vi "ConfigureRobot.vi"(8 "Pigeon Talon":T1, 9 "Pigeon":T6 {"Type" items=["CAN"=352321536, "TalonSRX"=33554432]}, 10 "Right Side":T1, 11 "Left Side":T1) -> (1 "Pigeon":T6 {"Type" items=["CAN"=352321536, "TalonSRX"=33554432]}, 2 "Right Side":T1, 3 "Left Side":T1)   [LabVIEW 2017]
uses:
  <vilib>/Rock Robotics/WPI/ThirdParty/Phoenix-LabVIEW/Pigeon IMU/CTRE_PigeonIMU_DeviceRef.ctl
  <vilib>/Rock Robotics/WPI/ThirdParty/Phoenix-LabVIEW/Pigeon IMU/CTRE_PigeonIMU_ConnectionType.ctl
  <vilib>/Rock Robotics/WPI/MotorControl/WPI_MotorControlDeviceRef.ctl
  <vilib>/Rock Robotics/WPI/MotorControl/WPI_MotorControlType.ctl
  <vilib>/Rock Robotics/SystemInterfaces/DIO/FPGA_DIOPWMChannel.ctl
  <vilib>/Rock Robotics/WPI/PWM/WPI_PWMDeadband.ctl
  <vilib>/Rock Robotics/SystemInterfaces/DIO/FPGA_DIOChannel.ctl
  <vilib>/Rock Robotics/WPI/ThirdParty/Phoenix-LabVIEW/Motor Controller/Controls/CTRE_Phoenix_MotorControl_FeedbackDevice.ctl
  <vilib>/Rock Robotics/WPI/ThirdParty/Phoenix-LabVIEW/Motor Controller/Controls/CTRE_Phoenix_MotorControl_RemoteSourceType.ctl
  <vilib>/Rock Robotics/WPI/ThirdParty/Phoenix-LabVIEW/Motor Controller/Controls/CTRE_Phoenix_MotorControl_SensorTermFeedbackDevice_Enhanced.ctl
  <vilib>/Rock Robotics/WPI/ThirdParty/Phoenix-LabVIEW/Motor Controller/Controls/CTRE_Phoenix_MotorControl_StatusFrameEnhanced.ctl
  <vilib>/Rock Robotics/WPI/ThirdParty/Phoenix-LabVIEW/Motor Controller/Controls/CTRE_Phoenix_MotorControl_NeutralMode.ctl
  <vilib>/Rock Robotics/WPI/ThirdParty/Phoenix-LabVIEW/Motor Controller/Controls/CTRE_Phoenix_MotorControl_ControlMode.ctl
  Constants.vi
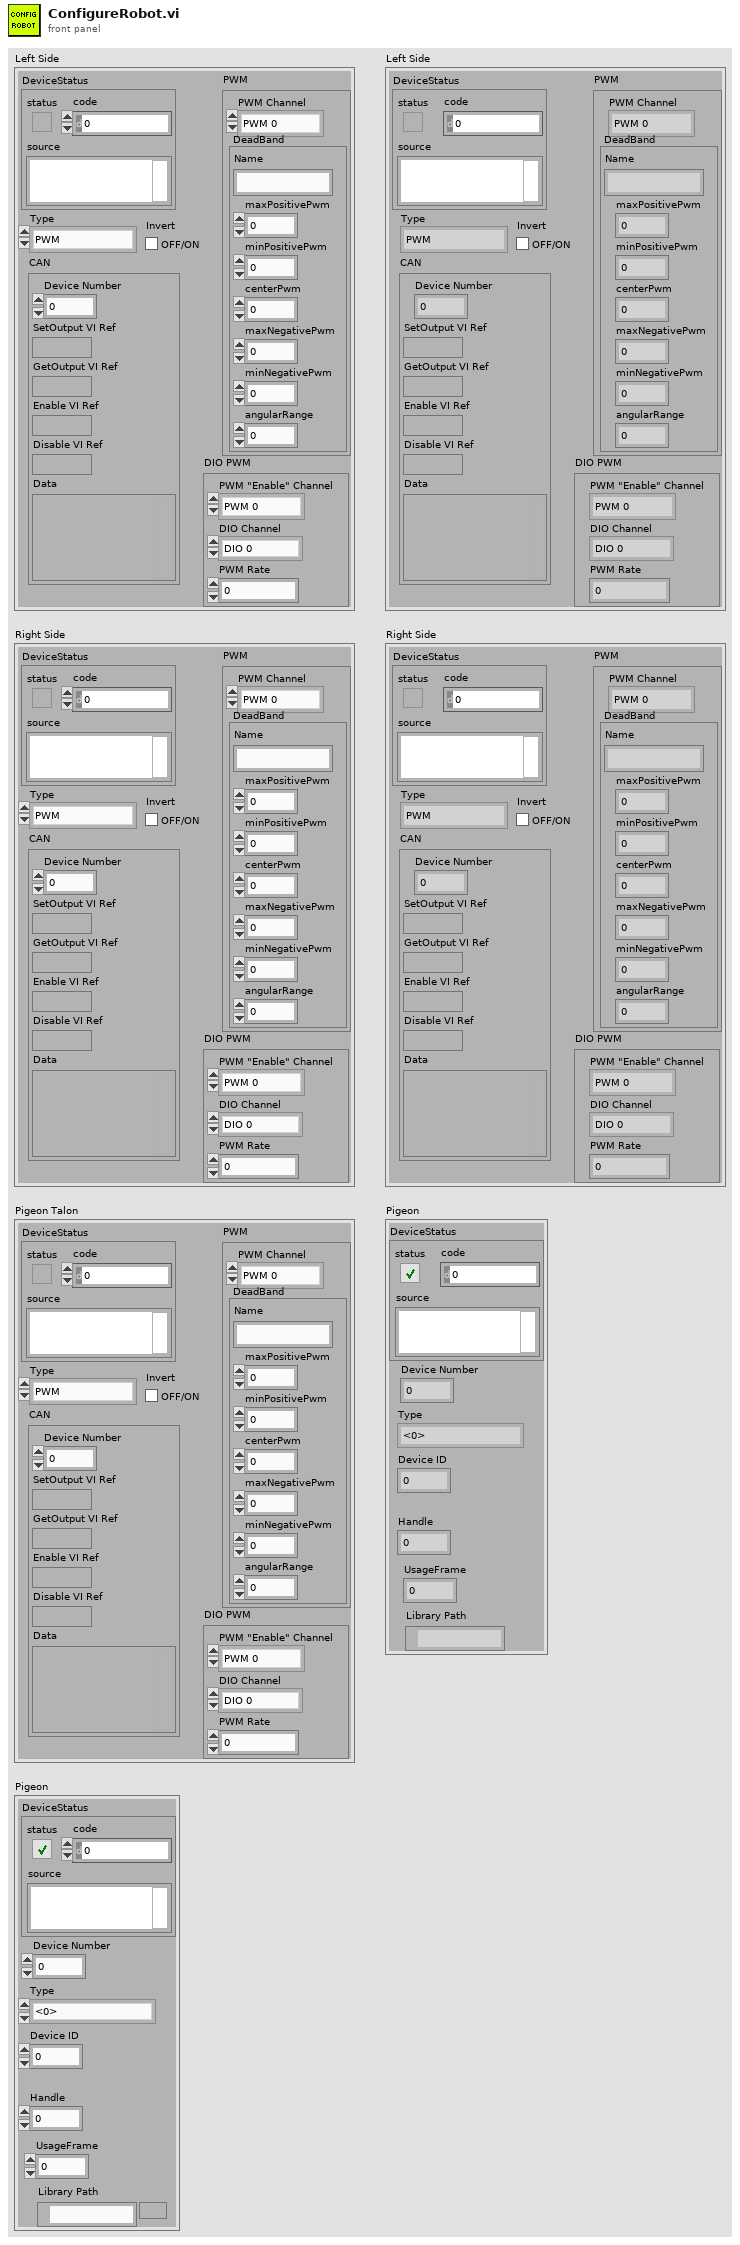
[diagram p1: front panel]
types:
  T1 = typedef "WPI_MotorControlDeviceRef.ctl" = cluster{"DeviceStatus":errorcluster, "Type":T2, "PWM":cluster{"PWM Channel":T3, "DeadBand":T4}, "CAN":cluster{"Device Number":u8, "SetOutput VI Ref":variant, "GetOutput VI Ref":variant, "Enable VI Ref":variant, "Disable VI Ref":variant, "Data":variant}, "Invert":bool, "DIO PWM":cluster{"PWM \"Enable\" Channel":T3, "DIOChannel":T5, "PWM Rate":dbl}}
  T2 = typedef "WPI_MotorControlType.ctl" = enum16{"PWM", "CAN", "DIO PWM"}
  T3 = typedef "FPGA_DIOPWMChannel.ctl" = enum8{"PWM 0", "PWM 1", "PWM 2", "PWM 3", "PWM 4", "PWM 5", "PWM 6", "PWM 7", "PWM 8", "PWM 9", "PWM MXP 0", "PWM MXP 1", "PWM MXP 2", "PWM MXP 3", "PWM MXP 4", "PWM MXP 5", "PWM MXP 6", "PWM MXP 7", "PWM MXP 8", "PWM MXP 9", "Invalid"}
  T4 = typedef "WPI_PWMDeadband.ctl" = cluster{"Name":string, "maxPositivePwm":i32, "minPositivePwm":i32, "centerPwm":i32, "maxNegativePwm":i32, "minNegativePwm":i32, "angularRange":u16}
  T5 = typedef "FPGA_DIOChannel.ctl" = enum8{"DIO 0", "DIO 1", "DIO 2", "DIO 3", "DIO 4", "DIO 5", "DIO 6", "DIO 7", "DIO 8", "DIO 9", "DIO MXP 0", "DIO MXP 1", "DIO MXP 2", "DIO MXP 3", "DIO MXP 4", "DIO MXP 5", "DIO MXP 6", "DIO MXP 7", "DIO MXP 8", "DIO MXP 9", "DIO MXP 10", "DIO MXP 11", "DIO MXP 12", "DIO MXP 13", "DIO MXP 14", "DIO MXP 15", "SPI Port CS1", "SPI Port CS2", "SPI Port CS3", "SPI Port MISO", "SPI Port MOSI", "Invalid"}
  T6 = typedef "CTRE_PigeonIMU_DeviceRef.ctl" = cluster{"DeviceStatus":errorcluster, "Device Number":u8, "Type":T7, "Device ID":u32, "Handle":u64, "UsageFrame":u32, "Library Path":path}
  T7 = typedef "CTRE_PigeonIMU_ConnectionType.ctl" = u32
  T8 = typedef "CTRE_Phoenix_MotorControl_ControlMode.ctl" = u16
  T9 = typedef "CTRE_Phoenix_MotorControl_NeutralMode.ctl" = enum8{"EEPROMSetting", "Override to Coast", "Override to Brake"}
  T10 = typedef "CTRE_Phoenix_MotorControl_StatusFrameEnhanced.ctl" = u16
  T11 = typedef "CTRE_Phoenix_MotorControl_FeedbackDevice.ctl" = i8
  T12 = typedef "CTRE_Phoenix_MotorControl_SensorTermFeedbackDevice_Enhanced.ctl" = i8
  T13 = typedef "CTRE_Phoenix_MotorControl_RemoteSourceType.ctl" = enum16{"Off", "Talon SRX Selected Sensor", "Pigeon IMU Yaw", "Pigeon IMU Pitch", "Pigeon IMU Roll", "CANifier Quadrature", "CANifier PWM Input 0", "CANifier PWM Input 1", "CANifier PWM Input 2", "CANifier PWM Input 3", "Gadgeteer Pigeon Yaw", "Gadgeteer Pigeon Pitch", "Gadgeteer Pigeon Roll"}
  T14 = cluster{"kP":dbl, "kI ":dbl, "kD":dbl, "kF":dbl, "I Zone":dbl, "Peak Out":dbl}
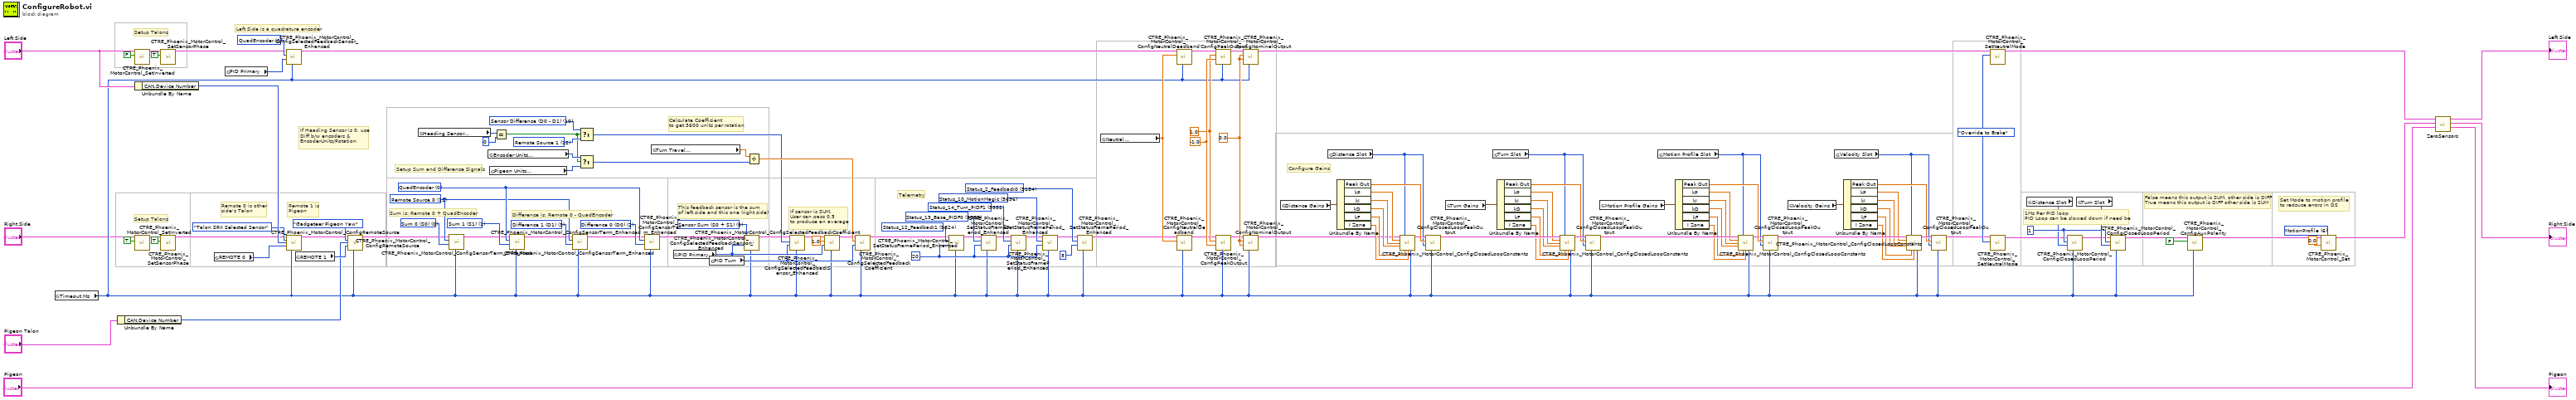
[diagram p0: block diagram]
diagram:
  w4 = T8 6 items=["PercentOutput"=0, "Position"=1, "Velocity"=2, "Current"=3, "Follower"=5, "MotionProfile"=6, "MotionMagic"=7, "MotionProfileArc"=10, "Disabled"=15] ("Control Mode")
  w123 = 1 ("loopTimeMs")
  w119 = CTRE_Phoenix_MotorControl_NeutralMode."Override to Brake" ("Motor Control Neutral Mode")
  w80 = 0.0 ("Forward Nominal Percent Output")
  w77 = -1.0 ("Reverse Peak Percent Output")
  w76 = 1.0 ("Forward Peak Percent Output")
  w69 = 20 ("periodMs")
  w68 = T10 5184 items=["Status_1_General"=5120, "Status_2_Feedback0"=5184, "Status_3_Quadrature"=5248, "Status_4_AinTempVbat"=5312, "Status_6_Misc"=5440, "Status_7_CommStatus"=5504, "Status_8_PulseWidth"=5568, "Status_9_MotProfBuffer"=5632, "Status_10_MotionMagic"=5696, "Status_11_UartGadgeteer"=5760, "Status_12_Feedback1"=5824, "Status_13_Base_PIDF0"=5888, "Status_14_Turn_PIDF1"=5952, "Status_15_FirmwareApiStatus"=6016] ("Status Frame")
  w67 = T10 5696 items=["Status_1_General"=5120, "Status_2_Feedback0"=5184, "Status_3_Quadrature"=5248, "Status_4_AinTempVbat"=5312, "Status_6_Misc"=5440, "Status_7_CommStatus"=5504, "Status_8_PulseWidth"=5568, "Status_9_MotProfBuffer"=5632, "Status_10_MotionMagic"=5696, "Status_11_UartGadgeteer"=5760, "Status_12_Feedback1"=5824, "Status_13_Base_PIDF0"=5888, "Status_14_Turn_PIDF1"=5952, "Status_15_FirmwareApiStatus"=6016] ("Status Frame")
  w66 = T10 5952 items=["Status_1_General"=5120, "Status_2_Feedback0"=5184, "Status_3_Quadrature"=5248, "Status_4_AinTempVbat"=5312, "Status_6_Misc"=5440, "Status_7_CommStatus"=5504, "Status_8_PulseWidth"=5568, "Status_9_MotProfBuffer"=5632, "Status_10_MotionMagic"=5696, "Status_11_UartGadgeteer"=5760, "Status_12_Feedback1"=5824, "Status_13_Base_PIDF0"=5888, "Status_14_Turn_PIDF1"=5952, "Status_15_FirmwareApiStatus"=6016] ("Status Frame")
  w65 = T10 5888 items=["Status_1_General"=5120, "Status_2_Feedback0"=5184, "Status_3_Quadrature"=5248, "Status_4_AinTempVbat"=5312, "Status_6_Misc"=5440, "Status_7_CommStatus"=5504, "Status_8_PulseWidth"=5568, "Status_9_MotProfBuffer"=5632, "Status_10_MotionMagic"=5696, "Status_11_UartGadgeteer"=5760, "Status_12_Feedback1"=5824, "Status_13_Base_PIDF0"=5888, "Status_14_Turn_PIDF1"=5952, "Status_15_FirmwareApiStatus"=6016] ("Status Frame")
  w64 = T10 5824 items=["Status_1_General"=5120, "Status_2_Feedback0"=5184, "Status_3_Quadrature"=5248, "Status_4_AinTempVbat"=5312, "Status_6_Misc"=5440, "Status_7_CommStatus"=5504, "Status_8_PulseWidth"=5568, "Status_9_MotProfBuffer"=5632, "Status_10_MotionMagic"=5696, "Status_11_UartGadgeteer"=5760, "Status_12_Feedback1"=5824, "Status_13_Base_PIDF0"=5888, "Status_14_Turn_PIDF1"=5952, "Status_15_FirmwareApiStatus"=6016] ("Status Frame")
  w49 = T11 12 items=["None"=-1, "QuadEncoder"=0, "Analog"=2, "Tachometer"=4, "Pulse Width Encoded Position"=8, "Sensor Sum (S0 + S1)"=9, "Sensor Difference (D0 - D1)"=10, "Remote Source 0"=11, "Remote Source 1"=12, "Software Emulated"=15] ("Feedback Device")
  w48 = T11 10 items=["None"=-1, "QuadEncoder"=0, "Analog"=2, "Tachometer"=4, "Pulse Width Encoded Position"=8, "Sensor Sum (S0 + S1)"=9, "Sensor Difference (D0 - D1)"=10, "Remote Source 0"=11, "Remote Source 1"=12, "Software Emulated"=15] ("Feedback Device")
  w42 = T11 9 items=["None"=-1, "QuadEncoder"=0, "Analog"=2, "Tachometer"=4, "Pulse Width Encoded Position"=8, "Sensor Sum (S0 + S1)"=9, "Sensor Difference (D0 - D1)"=10, "Remote Source 0"=11, "Remote Source 1"=12, "Software Emulated"=15] ("Feedback Device")
  w40 = u16 2 items=["Sum 0 (S0)", "Sum 1 (S1)", "Difference 0 (D0)", "Difference 1 (D1)"] ("Sensor Term")
  w39 = u16 3 items=["Sum 0 (S0)", "Sum 1 (S1)", "Difference 0 (D0)", "Difference 1 (D1)"] ("Sensor Term")
  w34 = u16 1 items=["Sum 0 (S0)", "Sum 1 (S1)", "Difference 0 (D0)", "Difference 1 (D1)"] ("Sensor Term")
  w38 = T12 0 items=["None"=-1, "QuadEncoder"=0, "Analog"=2, "Tachometer"=4, "Pulse Width Encoded Position"=8, "Remote Source 0"=11, "Remote Source 1"=12, "Software Emulated"=15] ("Feedback Device")
  w32 = u16 0 items=["Sum 0 (S0)", "Sum 1 (S1)", "Difference 0 (D0)", "Difference 1 (D1)"] ("Sensor Term")
  w37 = T12 11 items=["None"=-1, "QuadEncoder"=0, "Analog"=2, "Tachometer"=4, "Pulse Width Encoded Position"=8, "Remote Source 0"=11, "Remote Source 1"=12, "Software Emulated"=15] ("Feedback Device")
  w20 = T11 0 items=["None"=-1, "QuadEncoder"=0, "Analog"=2, "Tachometer"=4, "Pulse Width Encoded Position"=8, "Sensor Sum (S0 + S1)"=9, "Sensor Difference (D0 - D1)"=10, "Remote Source 0"=11, "Remote Source 1"=12, "Software Emulated"=15] ("Feedback Device")
  # "Set Mode to motion profile\nto redsuce errors in DS"
  # "False means this output is SUM, other side is DIFF\nTrue means this output is DIFF other side is SUM"
  # "1Ms Per PID loop\nPID Loop can be slowed down if need be"
  # "Configure Gains"
  # "Setup Talons"
  # "Telemetry"
  # "If sensor is SUM,\nUser can pass 0.5\nto produce an average"
  # "Calculate Coefficient\nto get 3600 units per rotation"
  # "If Heading Sensor is 0, use \nDiff b/w encoders &\nEncoderUnits/Rotation"
  # "This feedback sensor is the sum\nof left side and this one (right side)"
  # "Difference is: Remote 0 - QuadEncoder"
  # "Sum is: Remote 0 + QuadEncoder"
  # "Setup Sum and Difference Signals"
  # "Remote 1 is\nPigeon"
  # "Remote 0 is other\nside's Talon"
  # "Left Side is a quadrature encoder"
  # "Setup Talons"
  n1 = global read "Constants.vi" "Timeout Ms"() -> (w11:i32)
  n2 = Unbundle By Name("Pigeon Talon") -> ("CAN.Device Number"=w29:u8)
  n3 = Unbundle By Name("Left Side") -> ("CAN.Device Number"=w24:u8)
  n4 = call <vilib>:"CTRE_Phoenix_MotorControl_SetInverted.vi"("Invert?"=FALSE, "PhoenixMotorControlDevRef"="Left Side") -> ("PhoenixMotorControlDevRef"=w15:T1)  [unwired: 8 in, 1 out]
  n5 = call <vilib>:"CTRE_Phoenix_MotorControl_SetInverted.vi"("Invert?"=TRUE, "PhoenixMotorControlDevRef"="Right Side") -> ("PhoenixMotorControlDevRef"=w16:T1)  [unwired: 8 in, 1 out]
  n6 = call <vilib>:"CTRE_Phoenix_MotorControl_SetSensorPhase.vi"("PhaseSensor"=TRUE, "PhoenixMotorControlDevRef"=w15) -> ("PhoenixMotorControlDevRef"=w19:T1)  [unwired: 8 in, 1 out]
  n7 = call <vilib>:"CTRE_Phoenix_MotorControl_SetSensorPhase.vi"("PhaseSensor"=TRUE, "PhoenixMotorControlDevRef"=w16) -> ("PhoenixMotorControlDevRef"=w21:T1)  [unwired: 8 in, 1 out]
  n8 = global read "Constants.vi" "REMOTE 0"() -> (w25:i32)
  n9 = global read "Constants.vi" "PID Primary"() -> (w131:i32)
  n10 = call <vilib>:"CTRE_Phoenix_MotorControl_ConfigSelectedFeedbackSensor_Enhanced.vi"("timeoutMs"=w11, "pidLoopIdx"=w131, "Feedback Device"=w20, "PhoenixMotorControlDevRef"=w19) -> ("PhoenixMotorControlDevRef"=w73:T1)  [unwired: 6 in, 1 out]
  n11 = call <vilib>:"CTRE_Phoenix_MotorControl_ConfigRemoteSource.vi"("PhoenixMotorControlDevRef"=w21, "Remote Device Type"=CTRE_Phoenix_MotorControl_RemoteSourceType."Talon SRX Selected Sensor", "Remote Device ID"=w24, "Source Index (0/1)"=w25, "timeoutMs"=w11) -> ("PhoenixMotorControlDevRef"=w26:T1)  [unwired: 9 in, 1 out]
  n12 = global read "Constants.vi" "REMOTE 1"() -> (w30:i32)
  n13 = call <vilib>:"CTRE_Phoenix_MotorControl_ConfigRemoteSource.vi"("PhoenixMotorControlDevRef"=w26, "Remote Device Type"=CTRE_Phoenix_MotorControl_RemoteSourceType."Gadgeteer Pigeon Yaw", "Remote Device ID"=w29, "Source Index (0/1)"=w30, "timeoutMs"=w11) -> ("PhoenixMotorControlDevRef"=w31:T1)  [unwired: 9 in, 1 out]
  n14 = global read "Constants.vi" "Heading Sensor\nChoice"() -> (w43:i32)
  n15 = call <vilib>:"CTRE_Phoenix_MotorControl_ConfigSensorTerm_Enhanced.vi"("timeoutMs"=w11, "Sensor Term"=w32, "Feedback Device"=w37, "PhoenixMotorControlDevRef"=w31) -> ("PhoenixMotorControlDevRef"=w33:T1)  [unwired: 6 in, 1 out]
  n16 = global read "Constants.vi" "Encoder Units\nPer Rotation"() -> (w51:i32)
  n17 = global read "Constants.vi" "Pigeon Units\nPer Rotatoin"() -> (w50:i32)
  n18 = Equal?(x=w43, y=0) -> (x = y?=w45:bool)
  n19 = call <vilib>:"CTRE_Phoenix_MotorControl_ConfigSensorTerm_Enhanced.vi"("timeoutMs"=w11, "Sensor Term"=w34, "Feedback Device"=w38, "PhoenixMotorControlDevRef"=w33) -> ("PhoenixMotorControlDevRef"=w36:T1)  [unwired: 6 in, 1 out]
  n20 = call <vilib>:"CTRE_Phoenix_MotorControl_ConfigSensorTerm_Enhanced.vi"("timeoutMs"=w11, "Sensor Term"=w39, "Feedback Device"=w37, "PhoenixMotorControlDevRef"=w36) -> ("PhoenixMotorControlDevRef"=w35:T1)  [unwired: 6 in, 1 out]
  n21 = Select(t=w48, s=w45, f=w49) -> (s? t:f=w47:T11)
  n22 = Select(t=w51, s=w45, f=w50) -> (s? t:f=w56:i32)
  n23 = call <vilib>:"CTRE_Phoenix_MotorControl_ConfigSensorTerm_Enhanced.vi"("timeoutMs"=w11, "Sensor Term"=w40, "Feedback Device"=w38, "PhoenixMotorControlDevRef"=w35) -> ("PhoenixMotorControlDevRef"=w41:T1)  [unwired: 6 in, 1 out]
  n24 = global read "Constants.vi" "Turn Travel\nUnits Per Rotation"() -> (w57:dbl)
  n25 = global read "Constants.vi" "PID Primary"() -> (w130:i32)
  n26 = global read "Constants.vi" "PID Turn"() -> (w55:i32)
  n27 = call <vilib>:"CTRE_Phoenix_MotorControl_ConfigSelectedFeedbackSensor_Enhanced.vi"("timeoutMs"=w11, "pidLoopIdx"=w130, "Feedback Device"=w42, "PhoenixMotorControlDevRef"=w41) -> ("PhoenixMotorControlDevRef"=w46:T1)  [unwired: 6 in, 1 out]
  n28 = Divide(x=w57, y=w56) -> (x/y=w58:dbl)
  n29 = call <vilib>:"CTRE_Phoenix_MotorControl_ConfigSelectedFeedbackSensor_Enhanced.vi"("timeoutMs"=w11, "pidLoopIdx"=w55, "Feedback Device"=w47, "PhoenixMotorControlDevRef"=w46) -> ("PhoenixMotorControlDevRef"=w52:T1)  [unwired: 6 in, 1 out]
  n30 = call <vilib>:"CTRE_Phoenix_MotorControl_ConfigSelectedFeedbackCoefficient.vi"("timoutMs"=w11, "pidIdx"=w130, "coefficient"=1.0, "PhoenixMotorControlDevRef"=w52) -> ("PhoenixMotorControlDevRef"=w54:T1)  [unwired: 6 in, 1 out]
  n31 = call <vilib>:"CTRE_Phoenix_MotorControl_ConfigSelectedFeedbackCoefficient.vi"("timoutMs"=w11, "pidIdx"=w55, "coefficient"=w58, "PhoenixMotorControlDevRef"=w54) -> ("PhoenixMotorControlDevRef"=w59:T1)  [unwired: 6 in, 1 out]
  n32 = call <vilib>:"CTRE_Phoenix_MotorControl_SetStatusFramePeriod_Enhanced.vi"("timeoutMs"=w11, "periodMs"=w69, "Status Frame"=w64, "PhoenixMotorControlDevRef"=w59) -> ("PhoenixMotorControlDevRef"=w60:T1)  [unwired: 6 in, 1 out]
  n33 = call <vilib>:"CTRE_Phoenix_MotorControl_SetStatusFramePeriod_Enhanced.vi"("timeoutMs"=w11, "periodMs"=w69, "Status Frame"=w65, "PhoenixMotorControlDevRef"=w60) -> ("PhoenixMotorControlDevRef"=w61:T1)  [unwired: 6 in, 1 out]
  n34 = call <vilib>:"CTRE_Phoenix_MotorControl_SetStatusFramePeriod_Enhanced.vi"("timeoutMs"=w11, "periodMs"=w69, "Status Frame"=w66, "PhoenixMotorControlDevRef"=w61) -> ("PhoenixMotorControlDevRef"=w62:T1)  [unwired: 6 in, 1 out]
  n35 = call <vilib>:"CTRE_Phoenix_MotorControl_SetStatusFramePeriod_Enhanced.vi"("timeoutMs"=w11, "periodMs"=w69, "Status Frame"=w67, "PhoenixMotorControlDevRef"=w62) -> ("PhoenixMotorControlDevRef"=w63:T1)  [unwired: 6 in, 1 out]
  n36 = call <vilib>:"CTRE_Phoenix_MotorControl_SetStatusFramePeriod_Enhanced.vi"("timeoutMs"=w11, "periodMs"=5, "Status Frame"=w68, "PhoenixMotorControlDevRef"=w63) -> ("PhoenixMotorControlDevRef"=w71:T1)  [unwired: 6 in, 1 out]
  n37 = global read "Constants.vi" "Neutral\nDeadband"() -> (w74:dbl)
  n38 = call <vilib>:"CTRE_Phoenix_MotorControl_ConfigNeutralDeadband.vi"("timeoutMs"=w11, "Percent Deadband"=w74, "PhoenixMotorControlDevRef"=w73) -> ("PhoenixMotorControlDevRef"=w75:T1)  [unwired: 7 in, 1 out]
  n39 = call <vilib>:"CTRE_Phoenix_MotorControl_ConfigNeutralDeadband.vi"("timeoutMs"=w11, "Percent Deadband"=w74, "PhoenixMotorControlDevRef"=w71) -> ("PhoenixMotorControlDevRef"=w72:T1)  [unwired: 7 in, 1 out]
  n40 = call <vilib>:"CTRE_Phoenix_MotorControl_ConfigPeakOutput.vi"("timeoutMs"=w11, "Reverse Peak Percent Output"=w77, "Forward Peak Percent Output"=w76, "PhoenixMotorControlDevRef"=w75) -> ("PhoenixMotorControlDevRef"=w79:T1)  [unwired: 6 in, 1 out]
  n41 = call <vilib>:"CTRE_Phoenix_MotorControl_ConfigPeakOutput.vi"("timeoutMs"=w11, "Reverse Peak Percent Output"=w77, "Forward Peak Percent Output"=w76, "PhoenixMotorControlDevRef"=w72) -> ("PhoenixMotorControlDevRef"=w78:T1)  [unwired: 6 in, 1 out]
  n42 = call <vilib>:"CTRE_Phoenix_MotorControl_ConfigNominalOutput.vi"("timeoutMs"=w11, "Reverse Nominal Percent Output"=w80, "Forward Nominal Percent Output"=w80, "PhoenixMotorControlDevRef"=w79) -> ("PhoenixMotorControlDevRef"=w118:T1)  [unwired: 6 in, 1 out]
  n43 = call <vilib>:"CTRE_Phoenix_MotorControl_ConfigNominalOutput.vi"("timeoutMs"=w11, "Reverse Nominal Percent Output"=w80, "Forward Nominal Percent Output"=w80, "PhoenixMotorControlDevRef"=w78) -> ("PhoenixMotorControlDevRef"=w81:T1)  [unwired: 6 in, 1 out]
  n44 = global read "Constants.vi" "Distance Gains"() -> (w82:T14)
  n45 = global read "Constants.vi" "Distance Slot"() -> (w8:i32)
  n46 = Unbundle By Name(w82) -> ("Peak Out"=w89:dbl, "kP"=w83:dbl, "kI"=w84:dbl, "kD"=w85:dbl, "kF"=w86:dbl, "I Zone"=w87:dbl)
  n47 = call <vilib>:"CTRE_Phoenix_MotorControl_ConfigClosedLoopConstants.vi"("PhoenixMotorControlDevRef"=w81, "slotIdx"=w8, "P"=w83, "I"=w84, "D"=w85, "F"=w86, "I Zone"=w87, "timeoutMs"=w11) -> ("PhoenixMotorControlDevRef"=w88:T1)  [unwired: 6 in, 1 out]
  n48 = call <vilib>:"CTRE_Phoenix_MotorControl_ConfigClosedLoopPeakOutput.vi"("timoutMs"=w11, "slotIdx"=w8, "peakOutput"=w89, "PhoenixMotorControlDevRef"=w88) -> ("PhoenixMotorControlDevRef"=w114:T1)  [unwired: 6 in, 1 out]
  n49 = global read "Constants.vi" "Turn Gains"() -> (w97:T14)
  n50 = global read "Constants.vi" "Turn Slot"() -> (w7:i32)
  n51 = Unbundle By Name(w97) -> ("Peak Out"=w90:dbl, "kP"=w96:dbl, "kI"=w95:dbl, "kD"=w94:dbl, "kF"=w93:dbl, "I Zone"=w92:dbl)
  n52 = call <vilib>:"CTRE_Phoenix_MotorControl_ConfigClosedLoopConstants.vi"("PhoenixMotorControlDevRef"=w114, "slotIdx"=w7, "P"=w96, "I"=w95, "D"=w94, "F"=w93, "I Zone"=w92, "timeoutMs"=w11) -> ("PhoenixMotorControlDevRef"=w91:T1)  [unwired: 6 in, 1 out]
  n53 = call <vilib>:"CTRE_Phoenix_MotorControl_ConfigClosedLoopPeakOutput.vi"("timoutMs"=w11, "slotIdx"=w7, "peakOutput"=w90, "PhoenixMotorControlDevRef"=w91) -> ("PhoenixMotorControlDevRef"=w115:T1)  [unwired: 6 in, 1 out]
  n54 = global read "Constants.vi" "Motion Profile Gains"() -> (w98:T14)
  n55 = global read "Constants.vi" "Motion Profile Slot"() -> (w9:i32)
  n56 = Unbundle By Name(w98) -> ("Peak Out"=w105:dbl, "kP"=w99:dbl, "kI"=w100:dbl, "kD"=w101:dbl, "kF"=w102:dbl, "I Zone"=w103:dbl)
  n57 = call <vilib>:"CTRE_Phoenix_MotorControl_ConfigClosedLoopConstants.vi"("PhoenixMotorControlDevRef"=w115, "slotIdx"=w9, "P"=w99, "I"=w100, "D"=w101, "F"=w102, "I Zone"=w103, "timeoutMs"=w11) -> ("PhoenixMotorControlDevRef"=w104:T1)  [unwired: 6 in, 1 out]
  n58 = call <vilib>:"CTRE_Phoenix_MotorControl_ConfigClosedLoopPeakOutput.vi"("timoutMs"=w11, "slotIdx"=w9, "peakOutput"=w105, "PhoenixMotorControlDevRef"=w104) -> ("PhoenixMotorControlDevRef"=w116:T1)  [unwired: 6 in, 1 out]
  n59 = global read "Constants.vi" "Velocity Gains"() -> (w113:T14)
  n60 = global read "Constants.vi" "Velocity Slot"() -> (w6:i32)
  n61 = Unbundle By Name(w113) -> ("Peak Out"=w106:dbl, "kP"=w112:dbl, "kI"=w111:dbl, "kD"=w110:dbl, "kF"=w109:dbl, "I Zone"=w108:dbl)
  n62 = call <vilib>:"CTRE_Phoenix_MotorControl_ConfigClosedLoopConstants.vi"("PhoenixMotorControlDevRef"=w116, "slotIdx"=w6, "P"=w112, "I"=w111, "D"=w110, "F"=w109, "I Zone"=w108, "timeoutMs"=w11) -> ("PhoenixMotorControlDevRef"=w107:T1)  [unwired: 6 in, 1 out]
  n63 = call <vilib>:"CTRE_Phoenix_MotorControl_ConfigClosedLoopPeakOutput.vi"("timoutMs"=w11, "slotIdx"=w6, "peakOutput"=w106, "PhoenixMotorControlDevRef"=w107) -> ("PhoenixMotorControlDevRef"=w117:T1)  [unwired: 6 in, 1 out]
  n64 = call <vilib>:"CTRE_Phoenix_MotorControl_SetNeutralMode.vi"("Motor Control Neutral Mode"=w119, "PhoenixMotorControlDevRef"=w118) -> ("PhoenixMotorControlDevRef"=w125:T1)  [unwired: 8 in, 1 out]
  n65 = call <vilib>:"CTRE_Phoenix_MotorControl_SetNeutralMode.vi"("Motor Control Neutral Mode"=w119, "PhoenixMotorControlDevRef"=w117) -> ("PhoenixMotorControlDevRef"=w120:T1)  [unwired: 8 in, 1 out]
  n66 = global read "Constants.vi" "Distance Slot"() -> (w121:i32)
  n67 = call <vilib>:"CTRE_Phoenix_MotorControl_ConfigClosedLoopPeriod.vi"("timoutMs"=w11, "slotIdx"=w121, "loopTimeMs"=w123, "PhoenixMotorControlDevRef"=w120) -> ("PhoenixMotorControlDevRef"=w122:T1)  [unwired: 6 in, 1 out]
  n68 = global read "Constants.vi" "Turn Slot"() -> (w124:i32)
  n69 = call <vilib>:"CTRE_Phoenix_MotorControl_ConfigClosedLoopPeriod.vi"("timoutMs"=w11, "slotIdx"=w124, "loopTimeMs"=w123, "PhoenixMotorControlDevRef"=w122) -> ("PhoenixMotorControlDevRef"=w12:T1)  [unwired: 6 in, 1 out]
  n70 = call <vilib>:"CTRE_Phoenix_MotorControl_ConfigAuxPolarity.vi"("timeoutMs"=w11, "Invert"=FALSE, "PhoenixMotorControlDevRef"=w12) -> ("PhoenixMotorControlDevRef"=w2:T1)  [unwired: 8 in]
  n71 = call <vilib>:"CTRE_Phoenix_MotorControl_Set.vi"("Output"=0.0, "Control Mode"=w4, "PhoenixMotorControlDevRef"=w2) -> ("PhoenixMotorControlDevRef"=w1:T1)  [unwired: 7 in, 1 out]
  n72 = call "ZeroSensors.vi"("Pigeon"="Pigeon", "Talon 2"=w1, "Talon 1"=w125) -> ("Pigeon"=→"Pigeon":T6, "Talon 2"=→"Right Side":T1, "Talon 1"=→"Left Side":T1)  [unwired: 6 in]
